vi "Write File.vi"(8 "error in (no error)":errorcluster, 9 "Data":variant, 10 "datalog path (use dialog)":path, 11 "Reflective Memory File in":refnum<class "Reflective Memory File.lvclass">) -> (0 "error out":errorcluster)   [LabVIEW 2015, in "RefMem DMA Custom Device.lvlib" / "Reflective Memory File.lvclass"]
uses:
  Reflective Memory File.lvclass
  <vilib>/NI/NI VeriStand Custom Device Import and Export Tool/File Interface Class/File Interface.lvclass
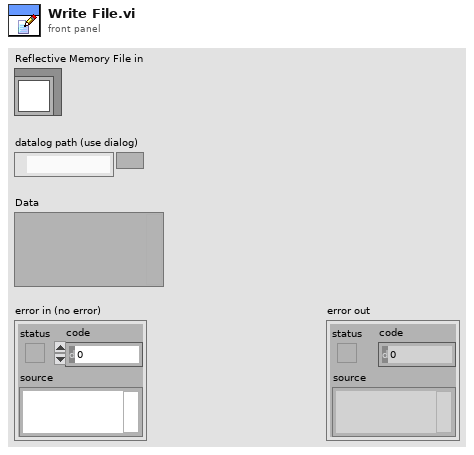
[diagram p1: front panel]
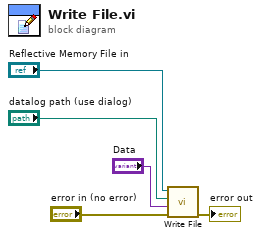
[diagram p0: block diagram]
diagram:
  n1 = call-parent "Write File.vi"("error in (no error)"="error in (no error)", "Data"="Data", "datalog path (use dialog)"="datalog path (use dialog)", "File Interface in"="Reflective Memory File in") -> ("error out"=→"error out":errorcluster)  [unwired: 7 in]
